vi "Write Ship_.vi"(8 "error in (no error)":errorcluster, 10 "Ship?":bool, 11 "Ship Wvfm Data MSG in":refnum<class "Ship Wvfm Data MSG.lvclass">) -> (0 "error out":errorcluster, 3 "Ship Wvfm Data MSG out":refnum<class "Ship Wvfm Data MSG.lvclass">)   [LabVIEW 2014, in "ePAS Library.lvlib" / "Ship Wvfm Data MSG.lvclass"]
uses:
  Ship Wvfm Data MSG.lvclass
  Ship Wvfm Data MSG.lvclass/Ship Wvfm Data MSG.ctl
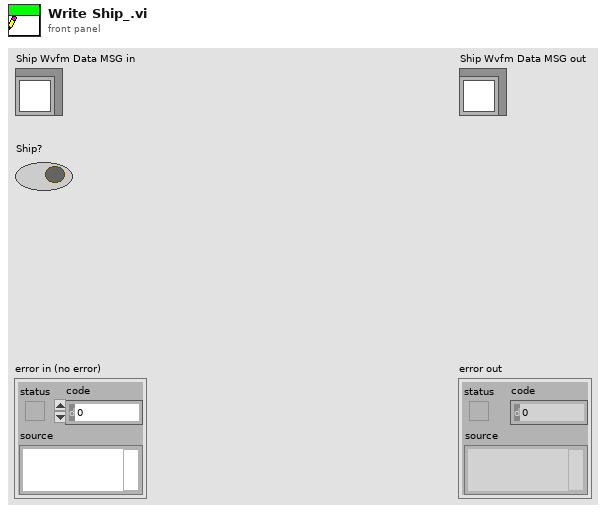
[diagram p1: front panel]
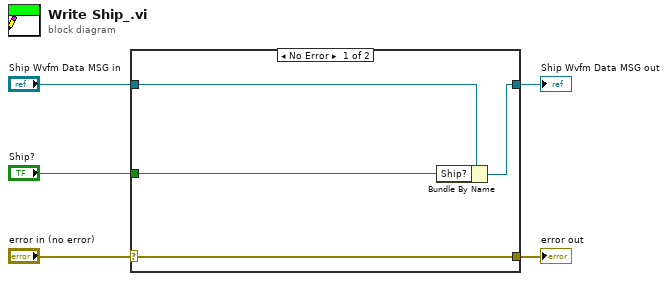
[diagram p0: block diagram]
diagram:
  n1 = case shown="No Error" "error in (no error)" {
    selector: "error in (no error)" -> [w9 w10]
    tunnel: [w9 w10] -> w4
    tunnel: [w7 w11] -> w2
    tunnel: "Ship Wvfm Data MSG in" -> [w8 w11]
    tunnel: "Ship?" -> [w6 _]
    frame No Error {
      n2 = Bundle By Name(cluster=w8, "Ship?"=w6) -> (w7:refnum<class "Ship Wvfm Data MSG.lvclass">)
    }
    frame Error {
    }
  }
  "error out" <- w4
  "Ship Wvfm Data MSG out" <- w2
